vi "Main.vi"   [LabVIEW 2017, in "Flightweight Pattern Demo.lvclass"]
uses:
  Flightweight Pattern Demo.lvclass
  ShapeFactory Class/fwShapeFactory.lvclass
  ConsoleOut/Print Options.ctl
  Flightweight Pattern Demo.lvclass/Flightweight Pattern Demo.ctl
  Circle Class/fwCircle.lvclass/fwCircle.ctl
  Circle Class/fwCircle.lvclass
types:
  T1 = typedef "Print Options.ctl" = enum16{"Create", "Get Reference", "Print", "Print Header", "Close"}
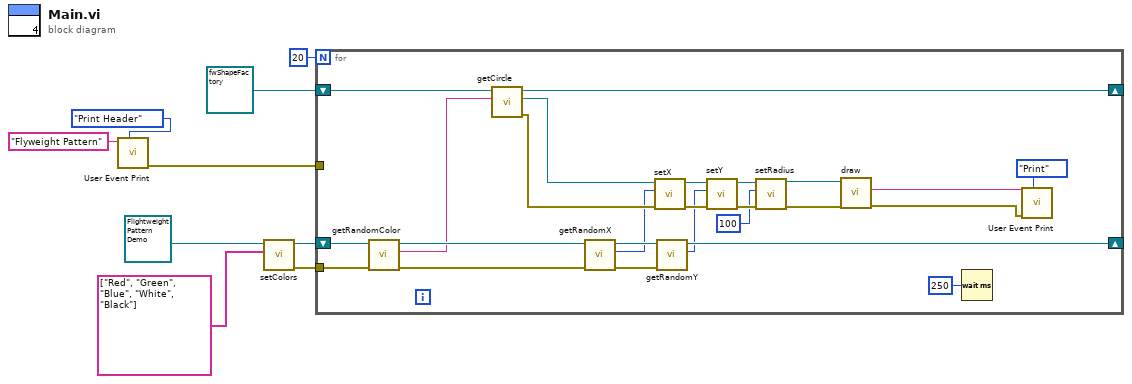
[diagram p0: block diagram]
diagram:
  n1 = call "User Event Print.vi"("Options"=Print_Options."Print Header", "String to Print"="Flyweight Pattern") -> ("error out"=w1:errorcluster)  [unwired: 8 in, 1 out]
  n2 = call "setColors.vi"("colors"=string[] ["Red", "Green", "Blue", "White", "Black"], "Flightweight Pattern Demo in"=refnum<class "Flightweight Pattern Demo.lvclass"> refnum ("Flightweight Pattern Demo.lvclass")) -> ("error out"=w5:errorcluster, "Flightweight Pattern Demo out"=w6:refnum<class "Flightweight Pattern Demo.lvclass">)  [unwired: 8 in]
  n3 = for {
    N: 20 -> [_]
    shift-right: [w30] -> _
    shift-left: w6 -> [w34]
    tunnel: w5 -> [w23]
    shift-right: [w14] -> _
    shift-left: refnum<class "fwShapeFactory.lvclass"> refnum ("fwShapeFactory.lvclass") -> [w13]
    tunnel: w1 -> [_]
    n4 = call "getRandomColor.vi"("error in (no error)"=w23, "Flightweight Pattern Demo in"=w34) -> ("error out"=w12:errorcluster, "Color"=w32:string, "Flightweight Pattern Demo out"=w33:refnum<class "Flightweight Pattern Demo.lvclass">)  [unwired: 7 in]
    n5 = call "getCircle.vi"("color"=w32, "fwShapeFactory in"=w13) -> ("error out"=w29:errorcluster, "fwCircle.lvclass"=w28:refnum<class "fwCircle.lvclass">, "fwShapeFactory out"=w14:refnum<class "fwShapeFactory.lvclass">)  [unwired: 7 in]
    n6 = call "getRandomX.vi"("error in (no error)"=w12, "Flightweight Pattern Demo in"=w33) -> ("error out"=w22:errorcluster, "X"=w21:i32, "Flightweight Pattern Demo out"=w31:refnum<class "Flightweight Pattern Demo.lvclass">)  [unwired: 7 in]
    n7 = call "setX.vi"("error in (no error)"=w29, "x"=w21, "fwCircle in"=w28) -> ("error out"=w27:errorcluster, "fwCircle out"=w26:refnum<class "fwCircle.lvclass">)  [unwired: 7 in]
    n8 = call "getRandomY.vi"("error in (no error)"=w22, "Flightweight Pattern Demo in"=w31) -> ("Y"=w20:i32, "Flightweight Pattern Demo out"=w30:refnum<class "Flightweight Pattern Demo.lvclass">)  [unwired: 7 in, 1 out]
    n9 = call "setY.vi"("error in (no error)"=w27, "y"=w20, "fwCircle in"=w26) -> ("error out"=w25:errorcluster, "fwCircle out"=w24:refnum<class "fwCircle.lvclass">)  [unwired: 7 in]
    n10 = call "setRadius.vi"("error in (no error)"=w25, "radius"=100, "fwCircle in"=w24) -> ("error out"=w17:errorcluster, "fwCircle out"=w18:refnum<class "fwCircle.lvclass">)  [unwired: 7 in]
    n11 = call-dynamic "draw.vi"("error in (no error)"=w17, "fwCircle in"=w18) -> ("error out"=w10:errorcluster, "Output"=w16:string)  [unwired: 7 in, 1 out]
    n12 = Wait (ms)(milliseconds to wait=u32 250) -> ()  [unwired: 1 out]
    n13 = call "User Event Print.vi"("Options"=Print_Options."Print", "error in (no error)"=w10, "String to Print"=w16) -> ()  [unwired: 7 in, 2 out]
  }
